vi "Icai 105 - Simultry6.vi"() -> ()   [LabVIEW 2010]
uses:
  <vilib>/Utility/error.llb/DialogType.ctl
  <vilib>/DAQmx/write.llb/DAQmx Write (Analog DBL 1Chan 1Samp).vi
  <vilib>/DAQmx/write.llb/DAQmx Write (Analog 1D Wfm NChan NSamp).vi
  <vilib>/DAQmx/write.llb/DAQmx Write (Digital 1D Bool 1Chan 1Samp).vi
  <vilib>/DAQmx/write.llb/DAQmx Write (Analog Wfm 1Chan NSamp).vi
  <vilib>/DAQmx/create/channels.llb/DAQmx Create Channel (AO-Voltage-Basic).vi
  <vilib>/daqmx/miscellaneous.llb/DAQmx Fill In Error Info.vi
  <vilib>/Waveform/WDTOps.llb/WDT Append Waveforms DBL.vi
  <vilib>/DAQmx/create/channels.llb/DAQmx Create Channel (DO-Digital Output).vi
  <vilib>/DAQmx/configure/timing.llb/DAQmx Timing (Sample Clock).vi
  <vilib>/measure/NI_MABase.lvlib
panel:
  in  "lines":tag="Dev1/port0/line3"
  in  "Rising Logic Output Chan":tag="Dev1/ao2"
  in  "Modulation Duration samples / 2":i32=150000
  out "Multiplier to arrive at Modulation # of samples":dbl=297.555285
  in  "Samples (1Ms/s)":i32=700000
  out "min value":dbl
  in  "Falling Logic Output Chan":tag="Dev1/ao1"
  in  "FM Waveform Channel":tag="Dev1/ao3"
  out "error out":errorcluster caption="error out (DAQ)"
  out "Mod":dbl=118572.0
  out "Numeric 2":dbl=3900000.0 format="%#_7g"
  out "Numeric":dbl=3900000.0 format="%#_7g"
  in  "CAI/ICAI":bool=TRUE
  in  "Pre-Trig Samples":ext=300.0 format="%.2f"
  out "?":dbl=579698.7113293351 format="%#_6f"
  in  "Fs":dbl=1000000.0
  out "#s":dbl=39524.02451426849
  in  "Time int":i32=30000
  in  "Sensitivity":u16(ring)=14 items=["2 nV/fA", "5 nV/fA", "10 nV/fA", "20 nV/fA", "50 nV/fA", "100 nV/fA", "200 nV/fA", "500 nV/fA", "1 uV/pA", "2 uV/pA", "5 uV/pA", "10 uV/pA", "20 uV/pA", "50 uV/pA", "100 uV/pA", "200 uV/pA", "500 uV/pA", "1 mV/nA", "2 mV/nA", "5 mV/nA", "10 mV/nA", "20 mV/nA", "50 mV/nA", "100 mV/nA", "200 mV/nA", "500 mV/nA", "1 V/uA"]
  in  "Detection Bandwidth":u16(ring)=7 items=["10 us/ 25 kHz", "30 us /8.33 kHz", "100 us/ 2.50 kHz", "300 us/ 833 Hz", "1 ms /250 Hz", "3 ms /83.3 Hz", "10 ms/ 25 Hz", "30 ms/ 8.33 Hz", "100 ms/ 2.50 Hz", "300 ms/ 0.833 Hz ", "1 s/ 0.250 Hz", "3 s/ 0.0833 Hz", "10 s/0.025 Hz"]
  in  "SR 830 GPIB Address":i32=8
  in  "Freq 2":dbl=1226.6 format="%_7g"
  out "Iterat #":dbl=10.0
  in  "Iteration":dbl=17.0
  in  "stop 2":bool
  in  "pulse":bool=TRUE
  in  "Start":ext=0.05
  out "?":waveform(dbl)[](graph)
  in  "amplitude 2":dbl=0.25 format="%0.2p"
  in  "?":T1(ring)
  in  "phase 2":dbl format="%.2p"
  in  "Offset 2":dbl=-0.0 format="%#_6p"
  in  "frequency 4":dbl=100.0 format="%0.2p"
  in  "sampling info 4":cluster{"Fs":dbl, "#s":dbl}={"Fs"=1000000.0, "#s"=2500.0} {"Fs" format="%.2p"}
  in  "?":T1(ring)=enum."Triangle Wave"
  in  "offset 4":dbl=-1.0 format="%0.2p"
  in  "phase 4":dbl=90.0 format="%.2p"
  in  "amplitude 4":dbl=1.0 format="%0.2p"
  in  "frequency 1":dbl=100.0 format="%0.2p"
  in  "amplitude 1":dbl=1.0 format="%0.2p"
  in  "sampling info 1":cluster{"Fs":dbl, "#s":dbl}={"Fs"=1000000.0, "#s"=2500.0} {"Fs" format="%.2p"}
  in  "?":T1(ring)=enum."Triangle Wave"
  in  "phase 1":dbl=-90.0 format="%.2p"
  in  "Offset 1":dbl format="%#_6p"
  in  "iterat":dbl=1.0
  out "CW":dbl=123571.0
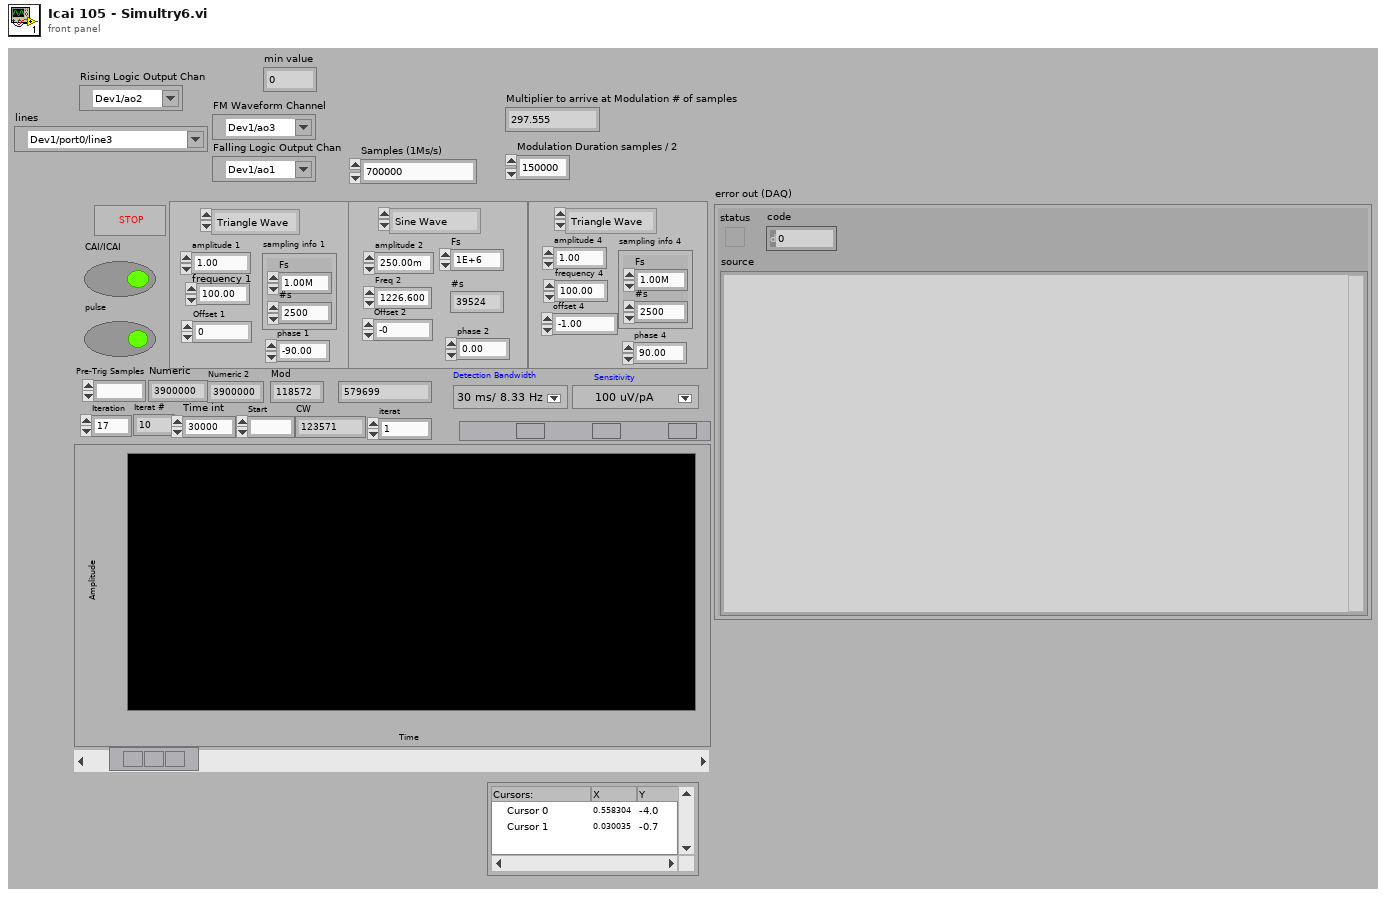
[diagram p1: front panel]
types:
  T1 = enum16{"Sine Wave", "Triangle Wave", "Square Wave", "Sawtooth Wave"}
  T2 = typedef "DialogType.ctl" = u16
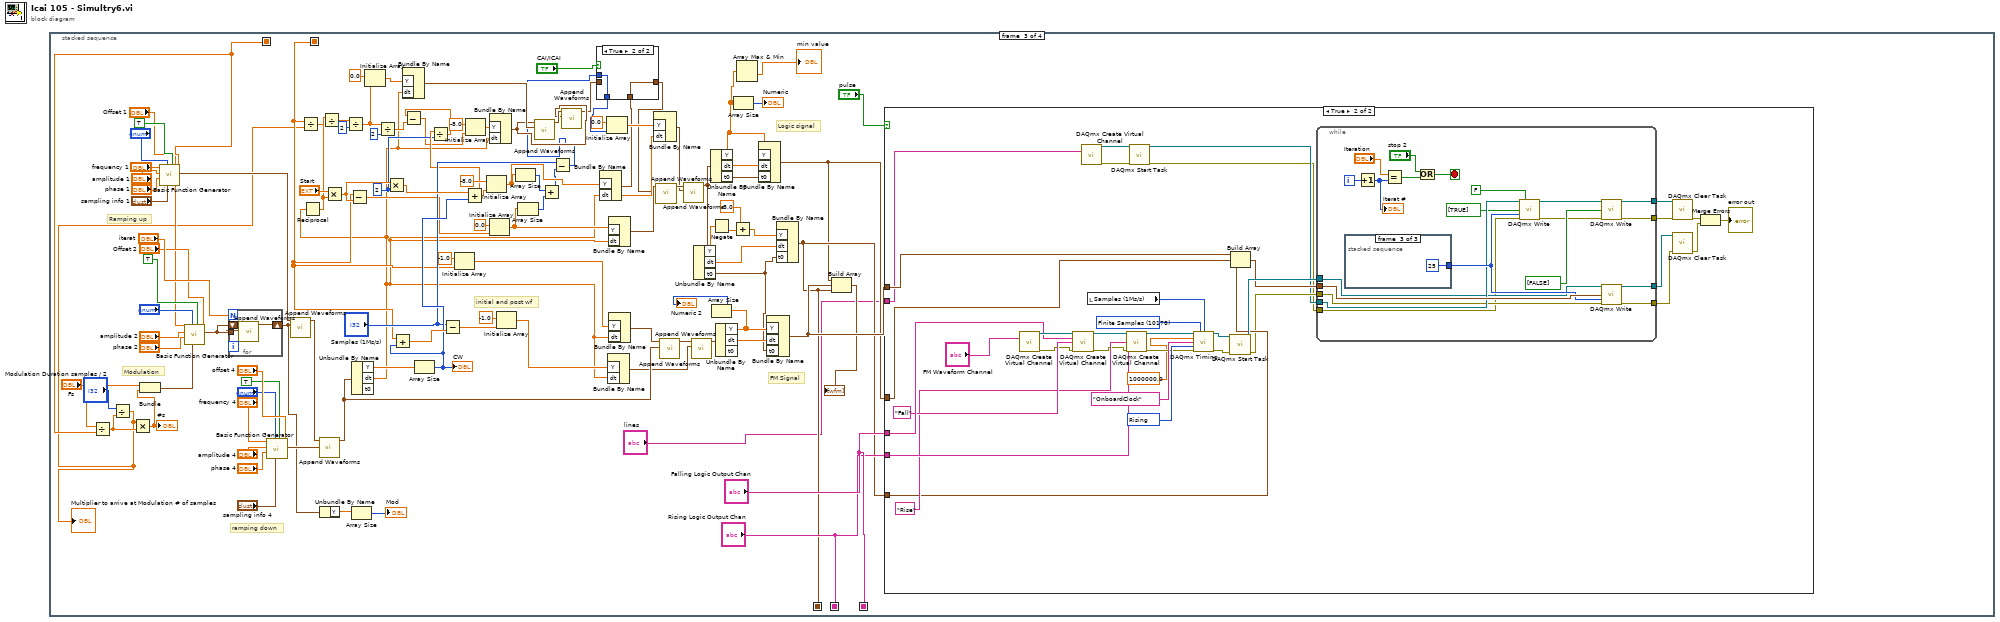
[diagram p0: block diagram]
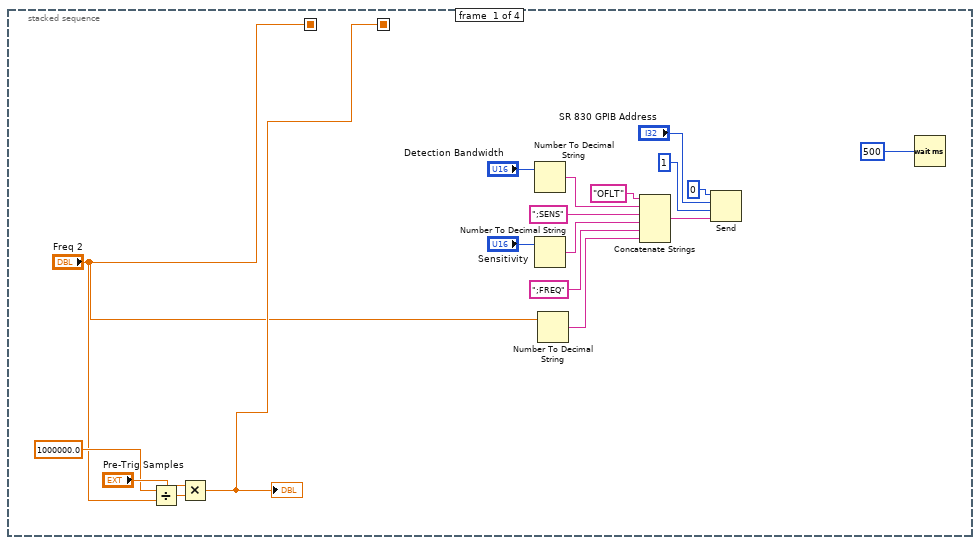
[diagram p2: hidden frame]
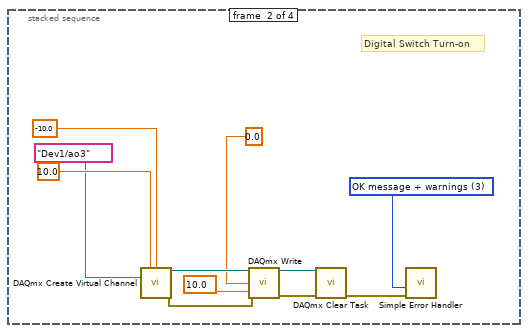
[diagram p3: hidden frame]
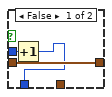
[diagram p4: hidden frame]
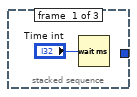
[diagram p6: hidden frame]
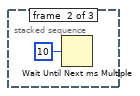
[diagram p7: hidden frame]
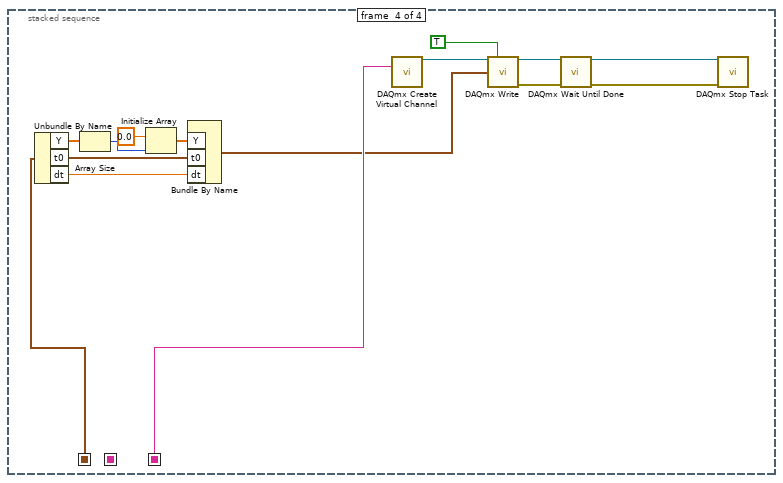
[diagram p8: hidden frame]
diagram:
  n1 = stacked-sequence {
    seq-local: ["Freq 2" _ _ _] -> [_ _ w85 _]
    seq-local: [w4 _ _ _] -> [_ _ w72 _]
    seq-local: [_ _ "Falling Logic Output Chan" _] -> [_ _ _ w212]
    seq-local: [_ _ "Rising Logic Output Chan" _] -> [_ _ _ _]
    seq-local: [_ _ w33 _] -> [_ _ _ w220]
    frame #0 {
      n2 = Divide(x=1000000.0 ("Fs 2"), y="Freq 2") -> (x/y=w7:dbl)
      n3 = Multiply(x="Pre-Trig Samples", y=w7) -> (x*y=w4:ext)
      "?" <- w4
      n4 = Number To Decimal String(number="Detection Bandwidth") -> (decimal integer string=w17:string)  [unwired: 1 out]
      n5 = Number To Decimal String(number="Sensitivity") -> (decimal integer string=w15:string)  [unwired: 1 out]
      n6 = Number To Decimal String(number="Freq 2") -> (decimal integer string=w2:string)  [unwired: 1 out]
      n7 = Concatenate Strings("OFLT", w17, ";SENS", w15, ";FREQ" ("string"), w2) -> (w14:string)
      n8 = Send(0:0 ("bus"), 2:"SR 830 GPIB Address", 3:i16 1 ("mode"), 5:w14) -> ()  [unwired: 1 in, 3 out]
      n9 = Wait (ms)(milliseconds to wait=500) -> ()  [unwired: 1 out]
    }
    frame #1 {
      w22 = T2 3 items=["no dialog", "OK message", "continue or stop message", "OK message + warnings", "continue/stop + warnings"] ("type of dialog (OK msg:1)")
      # "Digital Switch Turn-on"
      n10 = call-poly <vilib>:"DAQmx Create Virtual Channel.vi"("maximum value"=10.0 ("Maximum Value"), "minimum value"=-10.0 ("Minimum Value"), "physical channels"=tag "Dev1/ao3" ("Physical Channel")) -> ("task out"=w25:refnum<k21>, "error out"=w26:errorcluster)  [unwired: 6 in, 5 out]
      n11 = call-poly <vilib>:"DAQmx Write.vi"("task/channels in"=w25, "data"=0.0 ("Voltage Output"), "timeout"=10.0, "error in"=w26) -> ("task out"=w20:refnum<k21>, "error out"=w21:errorcluster)  [unwired: 1 in, 9 out]
      n12 = call <vilib>:"DAQmx Clear Task.vi"("task in"=w20, "error in"=w21) -> ("error out"=w19:errorcluster)  [unwired: 13 out]
      n13 = call <vilib>:"Simple Error Handler.vi"("type of dialog (OK msg:1)"=w22, "error in (no error)"=w19) -> ()  [unwired: 8 out]
    }
    frame #2 {
      w80 = 2
      # "initial and post wf"
      # "FM Signal"
      # "Logic signal"
      # "Ramping up"
      # "ramping down"
      # "Modulation"
      n14 = Divide(x="Fs", y=w85) -> (x/y=w46:dbl)
      n15 = Divide(x="Modulation Duration samples / 2", y=w46) -> (x/y=w45:dbl)
      "Multiplier to arrive at Modulation # of samples" <- w45
      n16 = Multiply(x=w45, y=w46) -> (x*y=w48:dbl)
      "#s" <- w48
      n17 = Bundle("Fs"="Fs", w48) -> (w83:cluster{"Fs":dbl, dbl})  [unwired: 1 out]
      n18 = call <vilib>:"Basic Function Generator.vi"("offset"="Offset 1", "reset signal"=TRUE, "sampling info"="sampling info 1", "signal type"="?", "phase"="phase 1", "amplitude"="amplitude 1", "frequency"="frequency 1") -> ("signal out"=w121:waveform(dbl))  [unwired: 2 in, 2 out]
      n19 = call <vilib>:"Basic Function Generator.vi"("offset"="Offset 2", "reset signal"=TRUE, "sampling info"=w83, "signal type"="?", "phase"="phase 2", "amplitude"="amplitude 2", "frequency"=w85) -> ("signal out"=w86:waveform(dbl))  [unwired: 2 in, 2 out]
      n20 = for {
        N: "iterat" -> [_]
        shift-right: [w210] -> w51
        shift-left: w86 -> [w208]
        tunnel: w86 -> [w209]
        n21 = call-poly <vilib>:"Append Waveforms.vi"("waveform B"=w209, "waveform A"=w208) -> ("waveform out"=w210:waveform(dbl))  [unwired: 1 in, 8 out]
      }
      n22 = call <vilib>:"Basic Function Generator.vi"("offset"="offset 4", "reset signal"=TRUE, "sampling info"="sampling info 4", "signal type"="?", "phase"="phase 4", "amplitude"="amplitude 4", "frequency"="frequency 4") -> ("signal out"=w126:waveform(dbl))  [unwired: 2 in, 2 out]
      n23 = call-poly <vilib>:"Append Waveforms.vi"("waveform B"=w51, "waveform A"=w121) -> ("waveform out"=w120:waveform(dbl))  [unwired: 1 in, 8 out]
      n24 = Divide(x=w72, y=w45) -> (x/y=w73:ext)
      n25 = call-poly <vilib>:"Append Waveforms.vi"("waveform B"=w126, "waveform A"=w120) -> ("waveform out"=w119:waveform(dbl))  [unwired: 1 in, 8 out]
      n26 = Unbundle By Name(w51) -> ("Y"=w52:dbl[])
      n27 = Array Size(array=w52) -> (size(s)=→"Mod":i32)
      n28 = Unbundle By Name(w119) -> ("Y"=w122:dbl[], "dt"=w64:dbl)  [unwired: 1 out]
      n29 = Reciprocal(x=w64) -> (1/x=w74:dbl)
      n30 = Divide(x=w74, y=w73) -> (x/y=w70:ext)
      n31 = Multiply(x="Start", y=w74) -> (x*y=w96:ext)
      n32 = Divide(x=w70, y=2) -> (x/y=w67:ext)
      n33 = Subtract(x=w72, y=w96) -> (x-y=w97:ext)
      n34 = Initialize Array(0.0 ("Trigger down"), w67) -> (w77:dbl[])
      n35 = Divide(x=w67, y=2) -> (x/y=w65:ext)
      n36 = Multiply(x=w96, y=w80) -> (x*y=w104:ext)
      n37 = Bundle By Name("Y"=w77, "dt"=w64) -> (w76:waveform(dbl))  [unwired: 1 out]
      n38 = Array Size(array=w122) -> (size(s)=w103:i32)
      "CW" <- w103
      n39 = Add(x=w72, y=w103) -> (x+y=w108:ext)
      n40 = Subtract(x="Samples (1Ms/s)", y=w108) -> (x-y=w107:ext)
      n41 = Initialize Array(-1.0 ("DC level"), w72) -> (w110:dbl[])
      n42 = Add(x=w104, y=w103) -> (x+y=w81:ext)
      n43 = Divide(x=w81, y=w80) -> (x/y=w69:ext)
      n44 = Subtract(x=w69, y=w65) -> (x-y=w68:ext)
      n45 = Initialize Array(-8.0 ("Trigger up"), w68) -> (w79:dbl[])
      n46 = Initialize Array(-8.0 ("Trigger up"), w81) -> (w94:dbl[])
      n47 = Bundle By Name("Y"=w79, "dt"=w64) -> (w63:waveform(dbl))  [unwired: 1 out]
      n48 = Initialize Array(0.0 ("Trigger down"), w97) -> (w95:dbl[])
      n49 = Initialize Array(-1.0 ("DC level"), w107) -> (w106:dbl[])
      n50 = Array Size(array=w94) -> (size(s)=w92:i32)
      n51 = Array Size(array=w95) -> (size(s)=w93:i32)
      n52 = call-poly <vilib>:"Append Waveforms.vi"("waveform B"=w76, "waveform A"=w63) -> ("waveform out"=w75:waveform(dbl))  [unwired: 1 in, 8 out]
      n53 = Add(x=w92, y=w93) -> (x+y=w91:i32)
      n54 = Subtract(x="Samples (1Ms/s)", y=w91) -> (x-y=w55:i32)
      n55 = call-poly <vilib>:"Append Waveforms.vi"("waveform B"=w63, "waveform A"=w75) -> ("waveform out"=w62:waveform(dbl))  [unwired: 1 in, 8 out]
      n56 = Bundle By Name("Y"=w94, "dt"=w64) -> (w60:waveform(dbl))  [unwired: 1 out]
      n57 = case shown="True" "CAI/ICAI" {
        tunnel: w62 -> [w145 _]
        tunnel: [w145 w147] -> w61
        tunnel: w60 -> [_ w147]
        tunnel: w55 -> [w144 w146]
        tunnel: [w143 w146] -> w54
        frame False {
          n58 = Increment(x=w144) -> (x+1=w143:i32)
        }
        frame True {
        }
      }
      n59 = Initialize Array(0.0 ("Trigger down"), w54) -> (w100:dbl[])
      n60 = Bundle By Name("Y"=w106, "dt"=w64) -> (w105:waveform(dbl))  [unwired: 1 out]
      n61 = Bundle By Name("Y"=w95, "dt"=w64) -> (w99:waveform(dbl))  [unwired: 1 out]
      n62 = Bundle By Name("Y"=w110, "dt"=w64) -> (w124:waveform(dbl))  [unwired: 1 out]
      n63 = Bundle By Name("Y"=w100, "dt"=w64) -> (w98:waveform(dbl))  [unwired: 1 out]
      n64 = call-poly <vilib>:"Append Waveforms.vi"("waveform B"=w61, "waveform A"=w99) -> ("waveform out"=w116:waveform(dbl))  [unwired: 1 in, 8 out]
      n65 = call-poly <vilib>:"Append Waveforms.vi"("waveform B"=w119, "waveform A"=w124) -> ("waveform out"=w125:waveform(dbl))  [unwired: 1 in, 8 out]
      n66 = call-poly <vilib>:"Append Waveforms.vi"("waveform B"=w98, "waveform A"=w116) -> ("waveform out"=w44:waveform(dbl))  [unwired: 1 in, 8 out]
      n67 = call-poly <vilib>:"Append Waveforms.vi"("waveform B"=w105, "waveform A"=w125) -> ("waveform out"=w113:waveform(dbl))  [unwired: 1 in, 8 out]
      n68 = Unbundle By Name(w44) -> ("Y"=w43:dbl[], "dt"=w38:dbl, "t0"=w39:timestamp)
      n69 = Unbundle By Name(w44) -> ("Y"=w50:dbl[], "dt"=w114:dbl, "t0"=w40:timestamp)
      n70 = Negate(x=w43) -> (-x=w41:dbl[])
      n71 = Unbundle By Name(w113) -> ("Y"=w56:dbl[], "dt"=w112:dbl)  [unwired: 1 out]
      n72 = Array Size(array=w56) -> (size(s)=→"Numeric 2":i32)
      n73 = Add(x=-8.0, y=w41) -> (x+y=w37:dbl[])
      n74 = Array Size(array=w50) -> (size(s)=→"Numeric":i32)
      n75 = Array Max & Min(array=w50) -> (min value=→"min value":dbl)  [unwired: 3 out]
      n76 = Bundle By Name("Y"=w50, "dt"=w114, "t0"=w40) -> (w32:waveform(dbl))  [unwired: 1 out]
      n77 = Bundle By Name("Y"=w56, "dt"=w112, "t0"=w39) -> (w49:waveform(dbl))  [unwired: 1 out]
      n78 = Bundle By Name("Y"=w37, "dt"=w38, "t0"=w39) -> (w33:waveform(dbl))  [unwired: 1 out]
      n79 = Build Array(w32, w49, w33) -> (→"?":waveform(dbl)[])
      n80 = case shown="True" "pulse" {
        tunnel: w49 -> [_ w166]
        tunnel: w32 -> [_ w165]
        tunnel: w33 -> [_ w164]
        tunnel: "Falling Logic Output Chan" -> [_ w181]
        tunnel: "Rising Logic Output Chan" -> [_ w178]
        tunnel: "lines" -> [_ w159]
        frame False {
        }
        frame True {
          w173 = 10178 items=["Finite Samples"=10178, "Continuous Samples"=10123, "Hardware Timed Single Point"=12522] ("sample mode")
          w174 = 10280 items=["Rising"=10280, "Falling"=10171] ("active edge")
          n81 = call-poly <vilib>:"DAQmx Create Virtual Channel.vi"("physical channels"="FM Waveform Channel") -> ("task out"=w182:refnum<k21>, "error out"=w168:errorcluster)  [unwired: 13 in]
          n82 = call-poly <vilib>:"DAQmx Create Virtual Channel.vi"("task in"=w182, "physical channels"=w181, "name to assign"="Fall", "error in"=w168) -> ("task out"=w179:refnum<k21>, "error out"=w169:errorcluster)  [unwired: 10 in]
          n83 = call-poly <vilib>:"DAQmx Create Virtual Channel.vi"("lines"=w159) -> ("task out"=w154:refnum<k21>, "error out"=w148:errorcluster)  [unwired: 13 in]
          n84 = local read "Samples (1Ms/s)"() -> (w155:i32)
          n85 = call-poly <vilib>:"DAQmx Create Virtual Channel.vi"("task in"=w179, "physical channels"=w178, "name to assign"="Rise", "error in"=w169) -> ("task out"=w176:refnum<k21>, "error out"=w170:errorcluster)  [unwired: 10 in]
          n86 = call <vilib>:"DAQmx Start Task.vi"("task/channels in"=w154, "error in"=w148) -> ("task out"=w158:refnum<k21>, "error out"=w157:errorcluster)  [unwired: 12 in]
          n87 = call-poly <vilib>:"DAQmx Timing.vi"("task/channels in"=w176, "sample mode"=w173, "samples per channel"=w155, "rate"=1000000.0, "source"=tag "OnboardClock", "active edge"=w174, "error in"=w170) -> ("task out"=w172:refnum<k21>, "error out"=w171:errorcluster)  [unwired: 7 in]
          n88 = call <vilib>:"DAQmx Start Task.vi"("task/channels in"=w172, "error in"=w171) -> ("task out"=w167:refnum<k21>, "error out"=w162:errorcluster)  [unwired: 12 in]
          n89 = Build Array(w166, w165, w164) -> (w163:waveform(dbl)[])
          n90 = while {
            tunnel: w167 -> [w193]
            tunnel: w163 -> [w198]
            tunnel: w162 -> [w192]
            tunnel: [w197] -> w160
            tunnel: [w196] -> w161
            tunnel: w158 -> [w194]
            tunnel: w157 -> [w190]
            tunnel: [w185] -> w152
            tunnel: [w184] -> w153
            i -> [w201]
            stop <- w202 stop-if-true
            n91 = stacked-sequence {
              tunnel: [_ _ 25 ("timeout (s)")] -> w195
              frame #0 {
                n92 = Wait (ms)(milliseconds to wait="Time int") -> ()  [unwired: 1 out]
              }
              frame #1 {
                n93 = Wait Until Next ms Multiple(millisecond multiple=u32 10) -> ()  [unwired: 1 out]
              }
              frame #2 {
              }
            }
            n94 = Increment(x=w201) -> (x+1=w199:i32)
            "Iterat #" <- w199
            n95 = Equal?(x="Iteration", y=w199) -> (x = y?=w204:bool)
            n96 = Or(x="stop 2", y=w204) -> (x .or. y?=w202:bool)
            n97 = call-poly <vilib>:"DAQmx Write.vi"("task/channels in"=w194, "auto start"=FALSE, "data"=bool[] [TRUE], "timeout"=w195, "error in"=w190) -> ("task out"=w188:refnum<k21>, "error out"=w186:errorcluster)  [unwired: 8 in, 1 out]
            n98 = call-poly <vilib>:"DAQmx Write.vi"("task/channels in"=w188, "data"=bool[] [FALSE], "error in"=w186) -> ("task out"=w184:refnum<k21>, "error out"=w185:errorcluster)  [unwired: 10 in, 1 out]
            n99 = call-poly <vilib>:"DAQmx Write.vi"("task/channels in"=w193, "data"=w198, "timeout"=w195, "error in"=w192) -> ("task out"=w197:refnum<k21>, "error out"=w196:errorcluster)  [unwired: 9 in, 1 out]
          }
          n100 = call <vilib>:"DAQmx Clear Task.vi"("task in"=w153, "error in"=w152) -> ("error out"=w151:errorcluster)  [unwired: 13 in]
          n101 = call <vilib>:"DAQmx Clear Task.vi"("task in"=w160, "error in"=w161) -> ("error out"=w149:errorcluster)  [unwired: 13 in]
          n102 = Merge Errors(w151, w149) -> (→"error out":errorcluster)
        }
      }
    }
    frame #3 {
      n103 = Unbundle By Name(w220) -> ("Y"=w217:dbl[], "t0"=w219:timestamp, "dt"=w218:dbl)
      n104 = Array Size(array=w217) -> (size(s)=w216:i32)
      n105 = Initialize Array(0.0 ("element"), w216) -> (w214:dbl[])
      n106 = Bundle By Name("Y"=w214, "t0"=w219, "dt"=w218) -> (w211:waveform(dbl))  [unwired: 1 in]
      n107 = call-poly <vilib>:"DAQmx Create Virtual Channel.vi"("physical channels"=w212) -> ("task out"=w213:refnum<k21>)  [unwired: 13 in, 1 out]
      n108 = call-poly <vilib>:"DAQmx Write.vi"("task/channels in"=w213, "auto start"=TRUE, "data"=w211) -> ("task out"=w221:refnum<k21>, "error out"=w224:errorcluster)  [unwired: 10 in, 1 out]
      n109 = call <vilib>:"DAQmx Wait Until Done.vi"("task/channels in"=w221, "error in"=w224) -> ("task out"=w223:refnum<k21>, "error out"=w225:errorcluster)  [unwired: 12 in]
      n110 = call <vilib>:"DAQmx Stop Task.vi"("task/channels in"=w223, "error in"=w225) -> ()  [unwired: 12 in, 2 out]
    }
  }
